vi "To Pythonic - Boolean Array.vi"(4 "Boolean Array":bool[](array[boolean])) -> (1 "Pythonic Value":string)   [LabVIEW 2016, in "OPI.lvclass"]
doc: "Convert LabVIEW data into valid pythonic representation."
uses:
  OPI.lvclass
  <vilib>/AdvancedString/Join Strings.vi
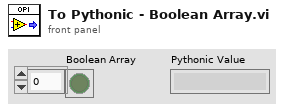
[diagram p1: front panel]
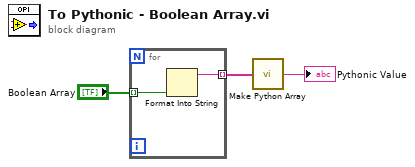
[diagram p0: block diagram]
diagram:
  n1 = for {
    tunnel: "Boolean Array" -> [w5] mode=indexing
    tunnel: [w4] -> w3 mode=indexing
    n2 = Format Into String(w5) -> (resulting string=w4:string)  [unwired: 3 in, 1 out]
  }
  n3 = call "Make Python Array.vi"("Pythonic Values"=w3) -> ("Pythonic Array"=→"Pythonic Value":string)
